vi "MH_WRabbitSetMode.vi"(7 "bootfromscript":i32, 8 "error in (no error)":errorcluster, 9 "mode":i32, 10 "reinit_with_mode":i32, 11 "devidx":i32) -> (0 "error out":errorcluster, 3 "return type":i32)   [LabVIEW 2019]
uses:
  MH_DllPath_global.vi
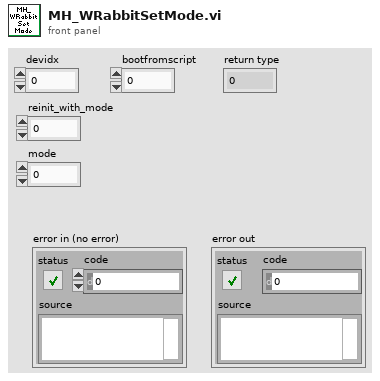
[diagram p1: front panel]
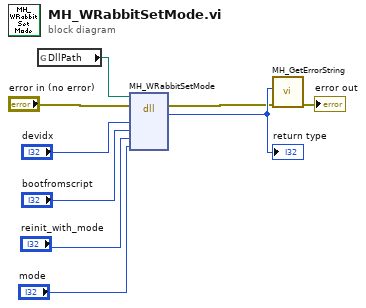
[diagram p0: block diagram]
diagram:
  n1 = global read "MH_DllPath_global.vi" "DllPath"() -> (w8:path)
  n2 = dll-call lib="mhlib64.dll" fn="MH_WRabbitSetMode"(path in=w8, error in="error in (no error)", "devidx"="devidx", "bootfromscript"="bootfromscript", "reinit_with_mode"="reinit_with_mode", "mode"="mode") -> (error out=w4:errorcluster, "return type"=w5:i32)  [unwired: 5 in, 1 out]
  "return type" <- w5
  n3 = call "MH_GetErrorString.vi"("error in (no error)"=w4, "code"=w5) -> ("error out"=→"error out":errorcluster)  [unwired: 7 in, 2 out]
